vi "ADC Delay Codification2.vi"(8 "Delay":dbl max=32767.0 step=1.0, 9 "ms/us Delay":bool) -> (0 "Final array":bool[](array[boolean]), 1 "Real Time":ext)   [LabVIEW 2011, in "NMR.lvclass"]
uses:
  NMR.lvclass
panel:
  out "Time Error":ext
  out "Aprox Loops":ext
  out "Pure Loops":ext
  in  "fixed-point type":fxp<+,15,15>
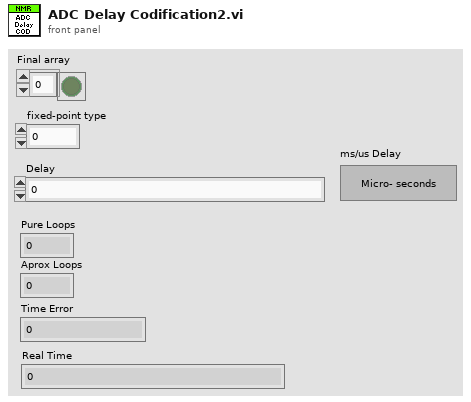
[diagram p1: front panel]
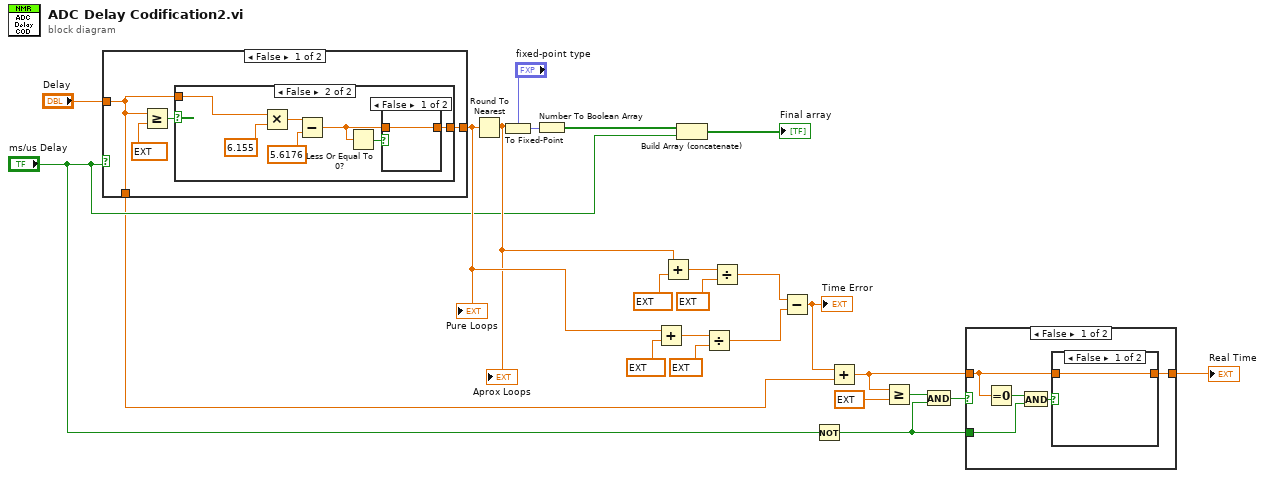
[diagram p0: block diagram]
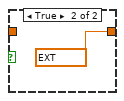
[diagram p2: hidden frame]
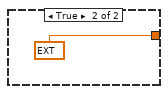
[diagram p3: hidden frame]
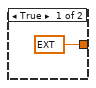
[diagram p4: hidden frame]
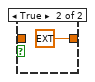
[diagram p5: hidden frame]
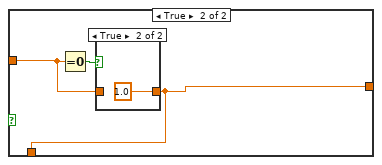
[diagram p6: hidden frame]
diagram:
  n1 = case shown="False" "ms/us Delay" {
    tunnel: "Delay" -> [w25 w40]
    tunnel: [w26 w39] -> w14
    tunnel: [w25 w39] -> w1
    frame False {
      n2 = Greater Or Equal?(x=w25, y=ext 1000.0) -> (x >= y?=w27:bool)
      n3 = case shown="False" w27 {
        tunnel: w25 -> [_ w36]
        tunnel: [ext 6149.0 w31] -> w26
        frame True {
        }
        frame False {
          n4 = Multiply(x=w36, y=6.155) -> (x*y=w34:dbl)
          n5 = Subtract(x=w34, y=5.6176) -> (x-y=w30:dbl)
          n6 = Less Or Equal To 0?(x=w30) -> (x <= 0?=w32:bool)
          n7 = case shown="False" w32 {
            tunnel: [w37 ext 0.0] -> w31
            tunnel: w30 -> [w37 _]
            frame False {
            }
            frame True {
            }
          }
        }
      }
    }
    frame True {
      n8 = Equal To 0?(x=w40) -> (x = 0?=w41:bool)
      n9 = case shown="True" w41 {
        tunnel: [w42 1.0] -> w39
        tunnel: w40 -> [w42 _]
        frame False {
        }
        frame True {
        }
      }
    }
  }
  "Pure Loops" <- w14
  n10 = Round To Nearest(number=w14) -> (nearest integer value=w11:ext)
  "Aprox Loops" <- w11
  n11 = To Fixed-Point(fixed-point type="fixed-point type", number=w11) -> (fixed-point=w23:fxp<+,15,15>)
  n12 = Number To Boolean Array(number=w23) -> (Boolean array=w22:bool[])
  n13 = Add(x=w14, y=ext 5.6176) -> (x+y=w16:ext)
  n14 = Add(x=w11, y=ext 5.6176) -> (x+y=w19:ext)
  n15 = Build Array (concatenate)(w22, "ms/us Delay") -> (→"Final array":bool[])
  n16 = Divide(x=w16, y=ext 6.1550000000000000002) -> (x/y=w12:ext)
  n17 = Divide(x=w19, y=ext 6.1550000000000000002) -> (x/y=w13:ext)
  n18 = Subtract(x=w13, y=w12) -> (x-y=w10:ext)
  "Time Error" <- w10
  n19 = Not(x="ms/us Delay") -> (.not. x?=w3:bool)
  n20 = Add(x=w10, y=w1) -> (x+y=w9:ext)
  n21 = Greater Or Equal?(x=w9, y=ext 1000.0) -> (x >= y?=w6:bool)
  n22 = And(x=w6, y=w3) -> (x .and. y?=w7:bool)
  n23 = case shown="False" w7 {
    tunnel: w9 -> [w45 _]
    tunnel: [w44 ext 1000.0] -> w4
    tunnel: w3 -> [w47 _]
    frame False {
      n24 = Equal To 0?(x=w45) -> (x = 0?=w48:bool)
      n25 = And(x=w48, y=w47) -> (x .and. y?=w46:bool)
      n26 = case shown="False" w46 {
        tunnel: w45 -> [w49 _]
        tunnel: [w49 ext 0.73746299999999999998] -> w44
        frame False {
        }
        frame True {
        }
      }
    }
    frame True {
    }
  }
  "Real Time" <- w4
